vi "SQL_test_template_name_select.vi"() -> (1 "error out":errorcluster, 3 "模板名称":string[][](table))   [LabVIEW 2014]
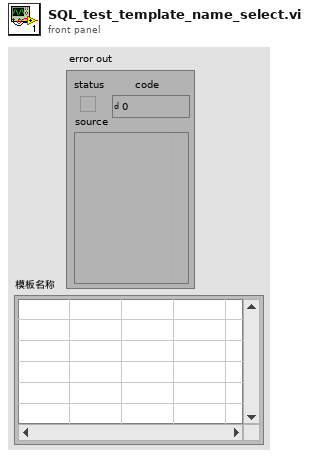
[diagram p1: front panel]
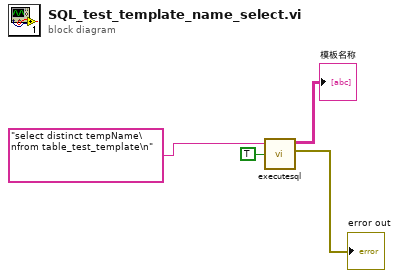
[diagram p0: block diagram]
diagram:
  n1 = call "executesql.vi"("Return Data (T)"=TRUE, "Command Text"="select distinct tempName\nfrom table_test_template\n") -> ("error out"=→"error out":errorcluster, "Data"=→"模板名称":string[][])  [unwired: 5 in]
